vi "TWM Client Cmd Start.vi"(5 "timeout [ms] (3000)":i32=3000, 7 "end of packet key":string="TWM:command:EndOfPacket", 8 "error in":errorcluster, 11 "handle":i32) -> (0 "error out":errorcluster, 3 "handle out":i32)   [LabVIEW 2020, in "TWM Client.lvlib"]
doc: "Write Start command packet to TWM server."
uses:
  TWM Client.lvlib
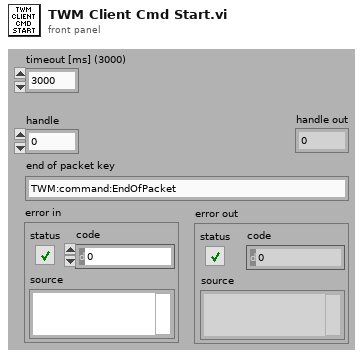
[diagram p1: front panel]
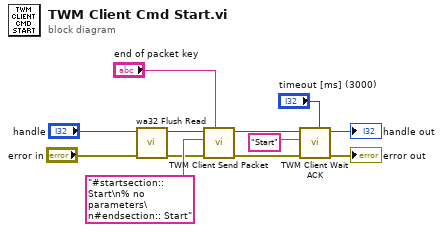
[diagram p0: block diagram]
diagram:
  n1 = call "wa32 Flush Read.vi"("error in"="error in", "handle"="handle") -> ("error out"=w3:errorcluster, "handle out"=w2:i32)  [unwired: 7 in, 1 out]
  n2 = call "TWM Client Send Packet.vi"("end of packet key"="end of packet key", "error in"=w3, "command string"="#startsection:: Start\n% no parameters\n#endsection:: Start", "handle"=w2) -> ("error out"=w10:errorcluster, "handle out"=w9:i32)  [unwired: 6 in]
  n3 = call "TWM Client Wait ACK.vi"("timeout [ms] (3000)"="timeout [ms] (3000)", "error in"=w10, "command header"="Start" ("key string"), "handle"=w9) -> ("error out"=→"error out":errorcluster, "handle out"=→"handle out":i32)  [unwired: 6 in]
